vi "Keithley DMM6500 DAQ6500 Series Mixed Function Scanning.vi"() -> ()   [LabVIEW 2023]
doc: "This example shows how to get mixed function scanning."
uses:
  <instrlib>/Keithley DMM6500 DAQ6500 Series/Public/Configure/Configure Temperature (Thermocouple).vi
  <instrlib>/Keithley DMM6500 DAQ6500 Series/Public/Data/Read (Multiple Points).vi
  <instrlib>/Keithley DMM6500 DAQ6500 Series/Keithley DMM6500 DAQ6500 Series.lvlib
panel:
  out "Measurements":dbl[](array[numeric])
  in  "Bandwidth (1: 30Hz)":i32(ring)=1 items=["3Hz", "30Hz", "300Hz"]
  in  "Thermocouple Type (3: K)":i32(ring)=3 items=["B", "E", "J", "K", "N", "R", "S", "T"]
  in  "Unit (1: Celsius)":i32(ring)=1 items=["Kelvin", "Celsius", "Fahrenheit"]
  in  "Reference Junction Type (1: Internal)":i32(ring)=1 items=["Simulated", "Internal", "External"]
  in  "Simulated Reference Temperature (0)":dbl
  in  "Delay Seconds (1 s)":dbl=1.0
  in  "Scan Count (1)":u32=1
  in  "VISA resource name":refnum<visa-resource-name>
  # "(c) 2018-2022 National Instruments.  ALL RIGHTS RESERVED."
  # "This example VI demonstrates how to use the DAQ6500 Series to perform complex multi-channel, mixed function scanning in a production-test environment."
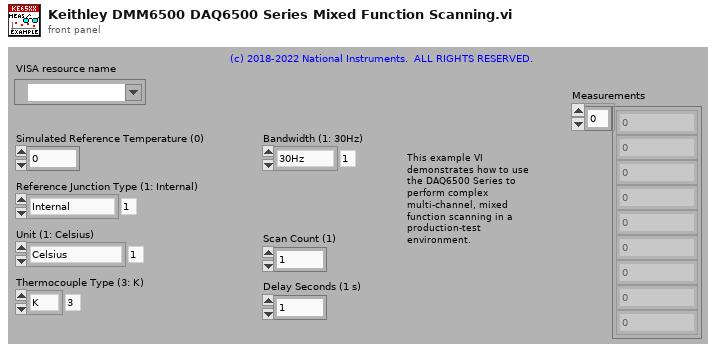
[diagram p1: front panel]
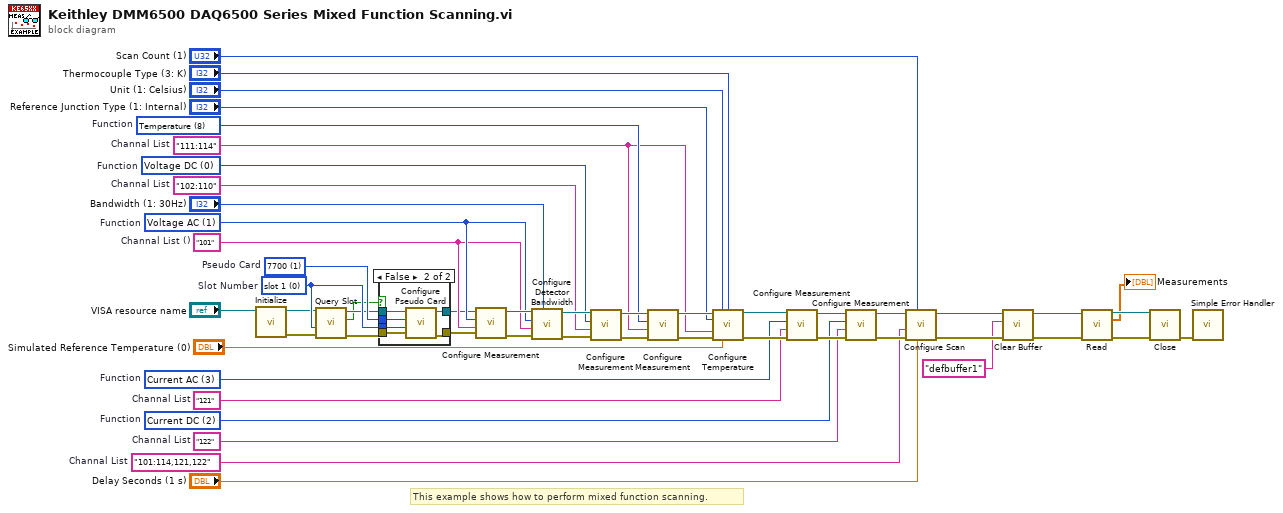
[diagram p0: block diagram]
diagram:
  w28 = "101:114,121,122"  # Channal List
  w20 = "122"  # Channal List
  w21 = 2 items=[" Voltage DC", "Voltage AC", "Current DC", "Current AC", "Resistance", "4-wire Resistance", "Diode", "Capacitance", "Temperature", "Continuity", "Frequency", "Period", "Voltage Ratio", "Digitize Voltage", "Digitize Current"]  # Function
  w22 = "121"  # Channal List
  w23 = 3 items=[" Voltage DC", "Voltage AC", "Current DC", "Current AC", "Resistance", "4-wire Resistance", "Diode", "Capacitance", "Temperature", "Continuity", "Frequency", "Period", "Voltage Ratio", "Digitize Voltage", "Digitize Current"]  # Function
  w38 = 8 items=[" Voltage DC", "Voltage AC", "Current DC", "Current AC", "Resistance", "4-wire Resistance", "Diode", "Capacitance", "Temperature", "Continuity", "Frequency", "Period", "Voltage Ratio", "Digitize Voltage", "Digitize Current"]  # Function
  w35 = "111:114"  # Channal List
  w41 = 0 items=[" Voltage DC", "Voltage AC", "Current DC", "Current AC", "Resistance", "4-wire Resistance", "Diode", "Capacitance", "Temperature", "Continuity", "Frequency", "Period", "Voltage Ratio", "Digitize Voltage", "Digitize Current"]  # Function
  w42 = "102:110"  # Channal List
  w25 = 1 items=[" Voltage DC", "Voltage AC", "Current DC", "Current AC", "Resistance", "4-wire Resistance", "Diode", "Capacitance", "Temperature", "Continuity", "Frequency", "Period", "Voltage Ratio", "Digitize Voltage", "Digitize Current"]  # Function
  w24 = "101"  # Channal List ()
  w8 = 0 items=["slot 1", "slot 2"]  # Slot Number
  w9 = 1 items=["0", "7700", "7701", "7702", "7703", "7705", "7706", "7707", "7708", "7709", "7710", "7711", "7712"]  # Pseudo Card
  # "This example shows how to perform mixed function scanning."
  n1 = call <instrlib>:"Initialize.vi"("VISA resource name"="VISA resource name") -> ("error out"=w6:errorcluster, "VISA resource name out"=w7:refnum<visa-resource-name>)  [unwired: 9 in]
  n2 = call <instrlib>:"Query Slot.vi"("error in (no error)"=w6, "Slot Number(0: slot 1)"=w8, "VISA resource name"=w7) -> ("error out"=w5:errorcluster, "Real Card In Slot"=w1:bool, "VISA resource name out"=w3:refnum<visa-resource-name>)  [unwired: 6 in]
  n3 = case shown="False" w1 {
    tunnel: w9 -> [_ w59]
    tunnel: w8 -> [_ w58]
    tunnel: w5 -> [w52 w57]
    tunnel: [w52 w56] -> w4
    tunnel: w3 -> [w53 w55]
    tunnel: [w53 w54] -> w2
    frame True {
    }
    frame False {
      n4 = call <instrlib>:"Configure Pseudo Card.vi"("error in (no error)"=w57, "Slot Number (0: slot1)"=w58, "Pseudo Card (0:No pseudocard)"=w59, "VISA resource name"=w55) -> ("error out"=w56:errorcluster, "VISA resource name out"=w54:refnum<visa-resource-name>)  [unwired: 6 in]
    }
  }
  n5 = call <instrlib>:"Configure Measurement.vi"("error in (no error)"=w4, "Channel List(\"\")"=w24, "Function (0: Voltage DC)"=w25, "VISA resource name"=w2) -> ("error out"=w45:errorcluster, "VISA resource name out"=w46:refnum<visa-resource-name>)  [unwired: 6 in]
  n6 = call <instrlib>:"Configure Detector Bandwidth.vi"("Bandwidth (1: 30Hz)"="Bandwidth (1: 30Hz)", "error in (no error)"=w45, "Channel List(\"\")"=w24, "Function (1: Voltage AC)"=w25, "VISA resource name"=w46) -> ("error out"=w43:errorcluster, "VISA resource name out"=w44:refnum<visa-resource-name>)  [unwired: 5 in]
  n7 = call <instrlib>:"Configure Measurement.vi"("error in (no error)"=w43, "Channel List(\"\")"=w42, "Function (0: Voltage DC)"=w41, "VISA resource name"=w44) -> ("error out"=w39:errorcluster, "VISA resource name out"=w40:refnum<visa-resource-name>)  [unwired: 6 in]
  n8 = call <instrlib>:"Configure Measurement.vi"("error in (no error)"=w39, "Channel List(\"\")"=w35, "Function (0: Voltage DC)"=w38, "VISA resource name"=w40) -> ("error out"=w36:errorcluster, "VISA resource name out"=w37:refnum<visa-resource-name>)  [unwired: 6 in]
  n9 = call-poly <instrlib>:"Configure Temperature.vi"("VISA resource name"=w37, "Unit (1: Celsius)"="Unit (1: Celsius)", "Thermocouple Type (3: K)"="Thermocouple Type (3: K)", "Reference Junction Type (1: Internal)"="Reference Junction Type (1: Internal)", "Channel List(\"\")"=w35, "error in (no error)"=w36, "Simulated Reference Temperature (0)"="Simulated Reference Temperature (0)") -> ("VISA resource name out"=w34:refnum<visa-resource-name>, "error out"=w33:errorcluster)  [unwired: 7 in]
  n10 = call <instrlib>:"Configure Measurement.vi"("error in (no error)"=w33, "Channel List(\"\")"=w22, "Function (0: Voltage DC)"=w23, "VISA resource name"=w34) -> ("error out"=w31:errorcluster, "VISA resource name out"=w32:refnum<visa-resource-name>)  [unwired: 6 in]
  n11 = call <instrlib>:"Configure Measurement.vi"("error in (no error)"=w31, "Channel List(\"\")"=w20, "Function (0: Voltage DC)"=w21, "VISA resource name"=w32) -> ("error out"=w29:errorcluster, "VISA resource name out"=w30:refnum<visa-resource-name>)  [unwired: 6 in]
  n12 = call <instrlib>:"Configure Scan.vi"("Delay Seconds (0 s)"="Delay Seconds (1 s)", "Scan Count (1)"="Scan Count (1)", "error in (no error)"=w29, "Channel List(\"\")"=w28, "VISA resource name"=w30) -> ("error out"=w18:errorcluster, "VISA resource name out"=w19:refnum<visa-resource-name>)  [unwired: 5 in]
  n13 = call <instrlib>:"Clear Buffer.vi"("error in (no error)"=w18, "Buffer Name (\"\")"="defbuffer1" ("Buffer Name ()"), "VISA resource name"=w19) -> ("error out"=w17:errorcluster, "VISA resource name out"=w16:refnum<visa-resource-name>)  [unwired: 7 in]
  n14 = call-poly <instrlib>:"Read.vi"("VISA resource name"=w16, "error in (no error)"=w17) -> ("VISA resource name out"=w48:refnum<visa-resource-name>, "Measurements"=→"Measurements":dbl[], "error out"=w49:errorcluster)  [unwired: 11 in]
  n15 = call <instrlib>:"Close.vi"("error in (no error)"=w49, "VISA resource name"=w48) -> ("error out"=w51:errorcluster)  [unwired: 9 in]
  n16 = call <vilib>:"Simple Error Handler.vi"("error in (no error)"=w51) -> ()  [unwired: 4 in, 5 out]
